vi "Pose_RelativeTo.vi"(9 "other POSE":T1, 11 "in POSE":T1) -> (3 "out POSE":T1)   [LabVIEW 2019, in "Trajectory_Library.lvlib"]
doc: "Returns the other pose relative to the current pose.\n\nThis function can often be used for trajectory tracking or pose stabilization algorithms to get the error between the reference and the current pose.\n\nParameters:\n - IN POSE - The POSE data structure\n - OTHER POSE - The pose that is the origin of the new coordinate frame that the current pose will be converted into.\n\nReturn:\n - OUT POSE - The current pose relative to the new origin pose."
uses:
  Trajectory_Library.lvlib
  POSE2D.ctl
  TRANSLATION2D.ctl
  ROTATION2D.ctl
  Rotation_UnaryMinus.vi
  Translation_RotateBy.vi
  Translation_Minus.vi
  Rotation_Minus.vi
  Rotation_CreateAngle.vi
  Translation_Create.vi
  Rotation_RotateBy.vi
  Rotation_CreateXY.vi
  Util_CalcDist.vi
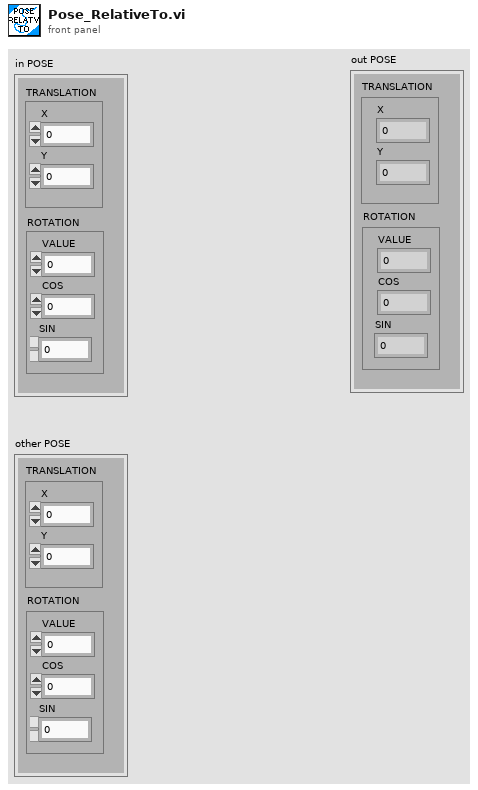
[diagram p1: front panel]
types:
  T1 = typedef "Trajectory_Library.lvlib/POSE2D.ctl" = cluster{"TRANSLATION":T2, "ROTATION":T3}
  T2 = typedef "Trajectory_Library.lvlib/TRANSLATION2D.ctl" = cluster{"X":dbl, "Y":dbl}
  T3 = typedef "Trajectory_Library.lvlib/ROTATION2D.ctl" = cluster{"VALUE":dbl, "COS":dbl, "SIN":dbl}
  T4 = typedef "Trajectory_Library.lvlib/TRANSFORM2D.ctl" = cluster{"TRANSLATION":T2, "ROTATION":T3}
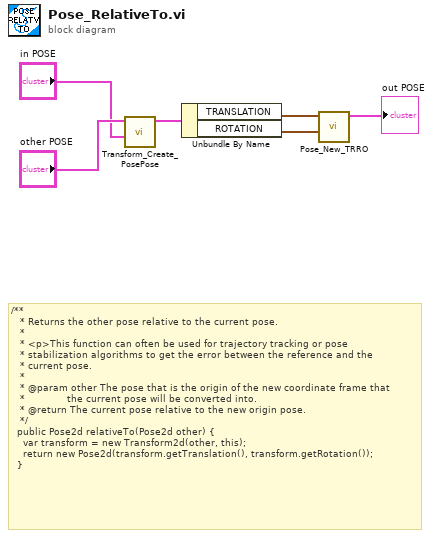
[diagram p0: block diagram]
diagram:
  # "/**\n   * Returns the other pose relative to the current pose.\n   *\n   * <p>This function can often be used for trajectory tracking or pose\n   * stabilization algorithms to get the error between the reference and the\n   * current pose.\n   *\n   * @param other The pose that is the origin of the new coordinate frame that\n   *              the current pose will be converted into.\n   * @return The current pose relative to the new origin pose.\n   */\n  public Pose2d relativeTo(Pose2d other) {\n    var transform = new Transform2d(other, this);\n    return new Pose2d(transform.getTranslation(), transform.getRotation());\n  }"
  n1 = call "Transform_Create_PosePose.vi"("last POSE"="in POSE", "initial POSE"="other POSE") -> ("TRANSFORM"=w6:T4)  [unwired: 9 in]
  n2 = Unbundle By Name(w6) -> ("TRANSLATION"=w2:T2, "ROTATION"=w1:T3)
  n3 = call "Pose_New_TRRO.vi"("ROTATION"=w1, "TRANSLATION"=w2) -> ("outPOSE"=→"out POSE":T1)  [unwired: 9 in]
